vi "test Change Between Specialty Digital And Non-Specialty Digital.vi"(8 "error in (no error)":errorcluster, 11 "TestCase in":refnum<class "Scan Engine cRIO System Tests.lvclass">) -> (0 "error out":errorcluster, 3 "TestCase out":refnum<class "Scan Engine cRIO System Tests.lvclass">)   [LabVIEW 2016, in "Scan Engine cRIO System Tests.lvclass"]
uses:
  Scan Engine cRIO System Tests.lvclass
  <vilib>/addons/_JKI Toolkits/VI Tester/TestCase.llb/TestCase.lvclass
  C:/Program Files (x86)/National Instruments/LabVIEW 2016/vi.lib/addons/_JKI Toolkits/VI Tester/TestCase.llb/TestCase.lvclass
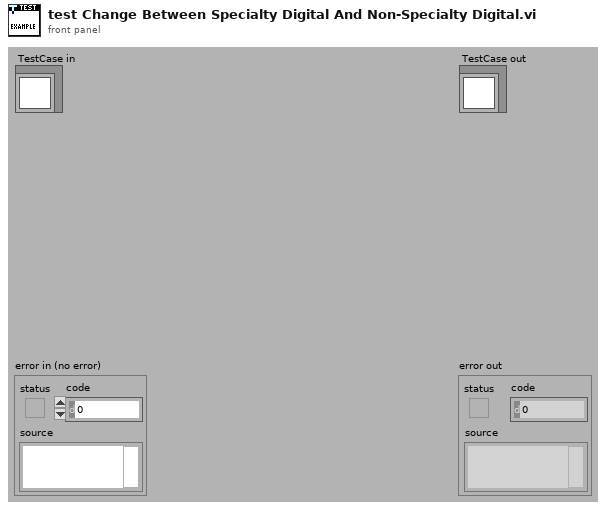
[diagram p1: front panel]
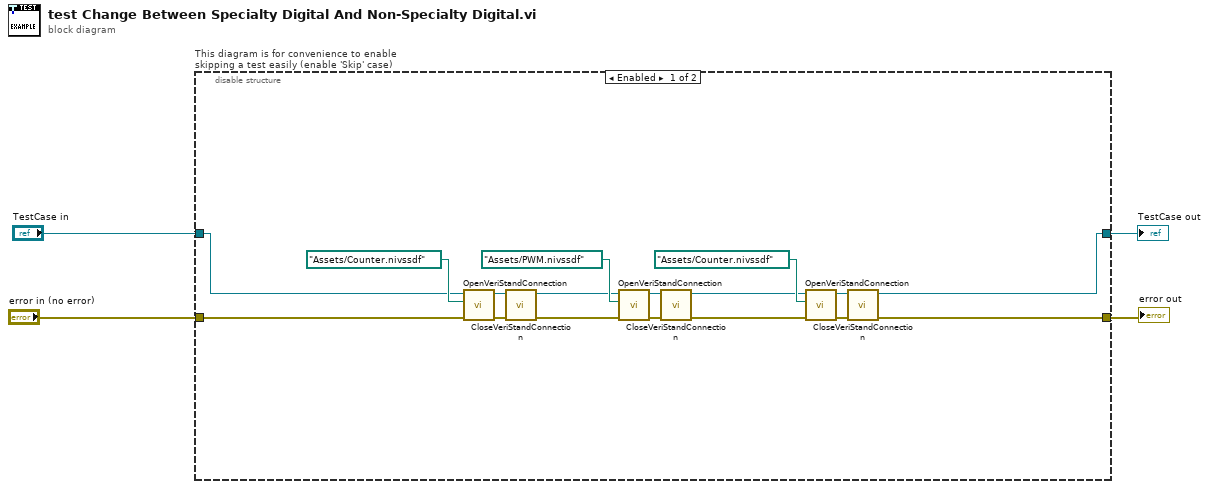
[diagram p0: block diagram]
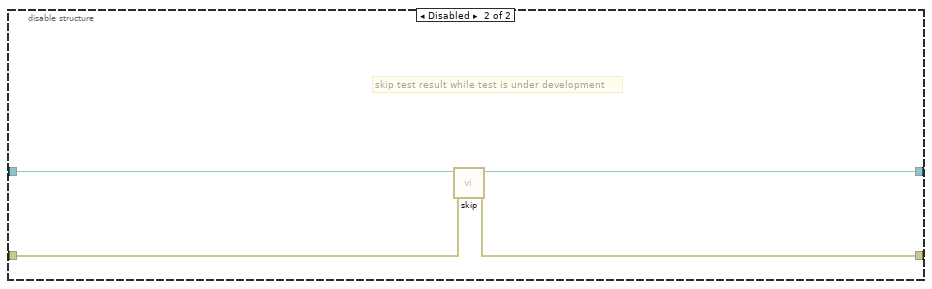
[diagram p2: hidden frame]
diagram:
  n1 = disable-structure "This diagram is for convenience to enable skipping a test easily (enable 'Skip' case)" shown="Enabled" {
    disable-tunnel: "TestCase in" -> [w19 w25]
    disable-tunnel: [w5 w23] -> w1
    disable-tunnel: [w6 w24] -> w3
    disable-tunnel: "error in (no error)" -> [w20 w22]
    frame Enabled {
      n2 = call-dynamic "OpenVeriStandConnection.vi"("error in (no error)"=w20, "System Definition File"=path "Assets/Counter.nivssdf", "VeriStand Test Case in"=w19) -> ("error out"=w18:errorcluster, "VeriStand Test Case out"=w17:refnum<class "Scan Engine cRIO System Tests.lvclass">)  [unwired: 7 in]
      n3 = call-dynamic "CloseVeriStandConnection.vi"("error in (no error)"=w18, "VeriStand Test Case in"=w17) -> ("error out"=w12:errorcluster, "VeriStand Test Case out"=w13:refnum<class "Scan Engine cRIO System Tests.lvclass">)  [unwired: 8 in]
      n4 = call-dynamic "OpenVeriStandConnection.vi"("error in (no error)"=w12, "System Definition File"=path "Assets/PWM.nivssdf", "VeriStand Test Case in"=w13) -> ("error out"=w15:errorcluster, "VeriStand Test Case out"=w14:refnum<class "Scan Engine cRIO System Tests.lvclass">)  [unwired: 7 in]
      n5 = call-dynamic "CloseVeriStandConnection.vi"("error in (no error)"=w15, "VeriStand Test Case in"=w14) -> ("error out"=w7:errorcluster, "VeriStand Test Case out"=w8:refnum<class "Scan Engine cRIO System Tests.lvclass">)  [unwired: 8 in]
      n6 = call-dynamic "OpenVeriStandConnection.vi"("error in (no error)"=w7, "System Definition File"=path "Assets/Counter.nivssdf", "VeriStand Test Case in"=w8) -> ("error out"=w10:errorcluster, "VeriStand Test Case out"=w11:refnum<class "Scan Engine cRIO System Tests.lvclass">)  [unwired: 7 in]
      n7 = call-dynamic "CloseVeriStandConnection.vi"("error in (no error)"=w10, "VeriStand Test Case in"=w11) -> ("error out"=w6:errorcluster, "VeriStand Test Case out"=w5:refnum<class "Scan Engine cRIO System Tests.lvclass">)  [unwired: 8 in]
    }
    frame Disabled {
      # "skip test result while test is under development"
      n8 = call <vilib>:"skip.vi"("error in (no error)"=w22, "TestCase in"=w25) -> ("error out"=w24:errorcluster, "TestCase out"=w23:refnum<class "Scan Engine cRIO System Tests.lvclass">)  [unwired: 8 in]
    }
  }
  "error out" <- w3
  "TestCase out" <- w1
